vi "Init.vi"(8 "error in (no error)":errorcluster, 9 "Constant Action Data":string, 10 "HAL GOOP4.lvlib:Instrument Base":refnum<class "Instrument.lvclass">, 11 "Virt Voltage Generator in":refnum<class "Virt Voltage Generator.lvclass">) -> (0 "error out":errorcluster, 3 "Virt Voltage Generator out":refnum<class "Virt Voltage Generator.lvclass">)   [LabVIEW 2023, in "Virt Instrs FGen.lvlib" / "Virt Voltage Generator.lvclass"]
uses:
  Virt Voltage Generator.lvclass
  Instrument/Instrument.lvclass
  Virtual Instrument Base/Virt Instr Base.lvclass
  Virt Voltage Generator.lvclass/Virt Voltage Generator.ctl
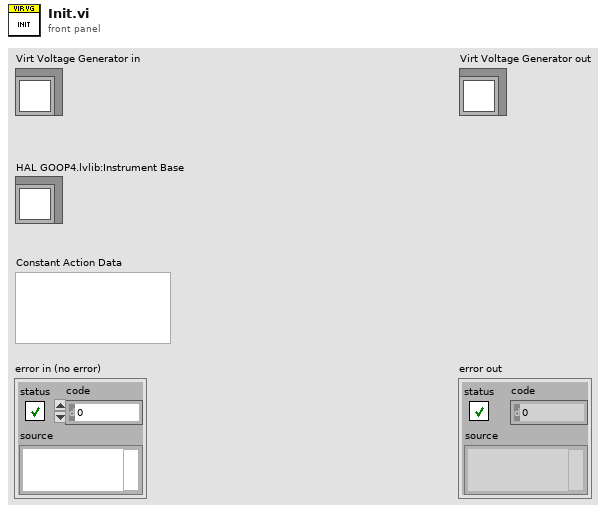
[diagram p1: front panel]
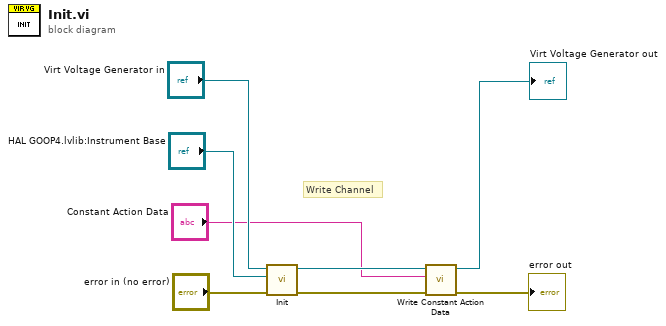
[diagram p0: block diagram]
diagram:
  # "Write Channel"
  n1 = call-parent "Init.vi"("error in (no error)"="error in (no error)", "HAL GOOP4.lvlib:Instrument"="HAL GOOP4.lvlib:Instrument Base", "Virt Instrument Base in"="Virt Voltage Generator in") -> ("error out"=w6:errorcluster, "Virt Instrument Base out"=w4:refnum<class "Virt Voltage Generator.lvclass">)  [unwired: 7 in]
  n2 = call "Write Constant Action Data.vi"("error in (no error)"=w6, "Constant Action Data"="Constant Action Data", "Virt Instrument Base in"=w4) -> ("error out"=→"error out":errorcluster, "Virt Instrument Base out"=→"Virt Voltage Generator out":refnum<class "Virt Voltage Generator.lvclass">)  [unwired: 7 in]
